vi "Process serial data.vi"(5 "Data in":string="SRNO=23234\nSOFT=40316\nXRT1=109\nSTAT=1089\nFREQ=170000\nSYNC=12345678\nEPOS=0\nDPOS=0\nINFO=2\nTIME=8427") -> (0 "Stage types":string[][](array[string]), 1 "Values":i32[](array[numeric]), 2 "Parameters":T1[](array[typedef]), 3 "Drive letters":string[](array[string]))   [LabVIEW 2019]
uses:
  Class/Controller/Serial parameters.ctl
  Class/Controller/Controller.lvclass
panel:
  out "array":string[](array[string])
  # "Example data single axis"
  # "Example data multi axis"
  # "SRNO=23234\nSOFT=40316\nXRT1=109\nSTAT=1089\nFREQ=170000\nSYNC=12345678\nEPOS=0\nDPOS=0\nINFO=2\nTIME=8427"
  # "A:SRNO=0\nA:SOFT=40305\nA:XLS1=313\nA:STAT=17\nA:FREQ=170000\nA:SYNC=12345678\nA:EPOS=2\nA:DPOS=0\nA:PHAC=0\nA:TIME=55599\nB:SRNO=0\nB:SOFT=40305\nB:XLA1=312\nB:STAT=17\nB:FREQ=173000\nB:SYNC=12345678\nB:EPOS=1\nB:DPOS=0\nB:PROP=120\nB:TIME=29533\nC:SRNO=0\nC:SOFT=40305\nC:XRT1=109\nC:STAT=1\nC:FREQ=173000\nC:SYNC=12345678\nC:EPOS=0\nC:DPOS=0\nC:PROP=120\nC:TIME=30364\nD:SRNO=0\nD:SOFT=40305\nD:XLS3=1251\nD:STAT=401\nD:FREQ=87000\nD:SYNC=12345678\nD:EPOS=0\nD:DPOS=0\nD:PROP=120\nD:TIME=30387\nE:SRNO=0\nE:SOFT=40305\nE:XLA3=1250\nE:STAT=17\nE:FREQ=87000\nE:SYNC=12345678\nE:EPOS=0\nE:DPOS=0\nE:PROP=120\nE:TIME=30355"
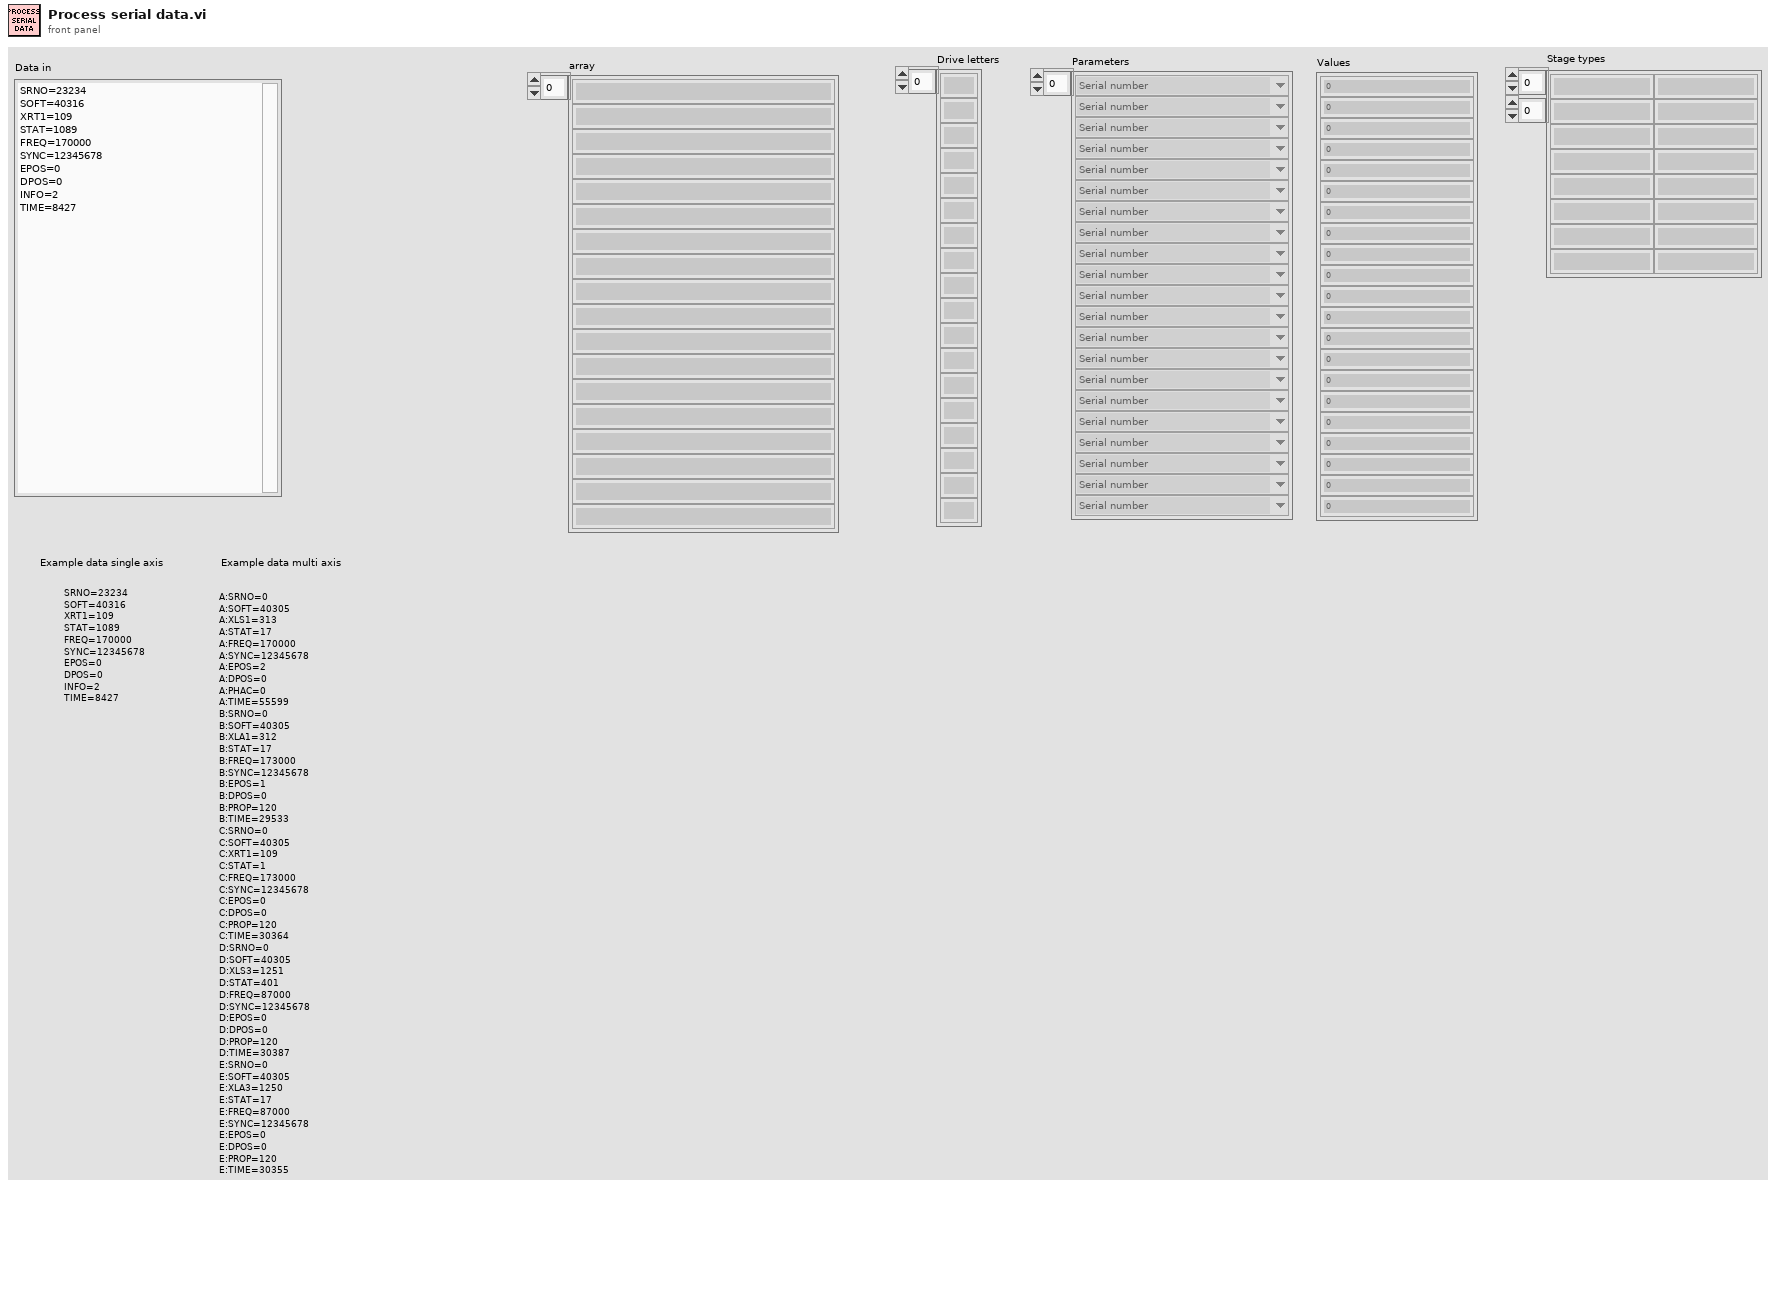
[diagram p1: front panel]
types:
  T1 = typedef "Controller.lvclass/Serial parameters.ctl" = enum16{"Serial number", "Software number", "Type of stage", "Status", "Frequency", "Encoder position", "Desired position", "Info", "Phase correction", "Timestamp", "Proportional control factor", "Sync", "XRT1", "XRT3", "XRTA", "XLS1", "XLS3", "XLA1", "XLA3"}
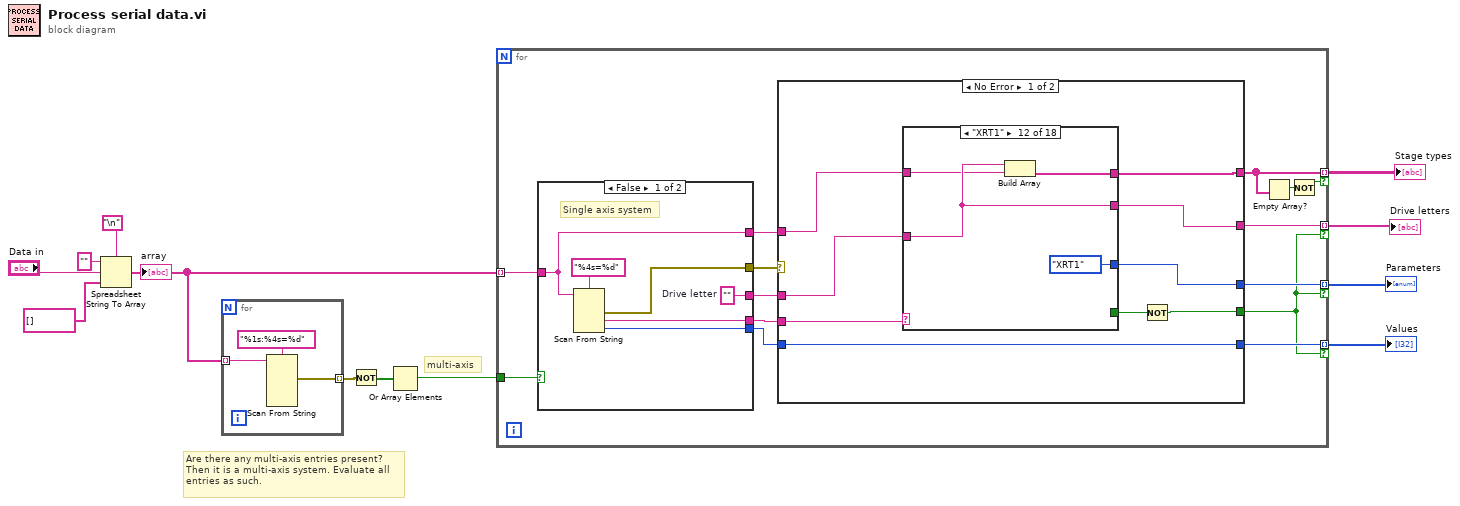
[diagram p0: block diagram]
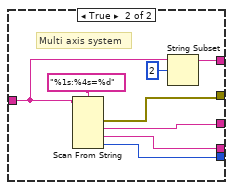
[diagram p2: hidden frame]
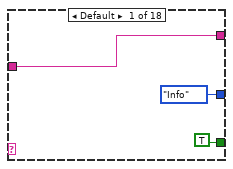
[diagram p3: hidden frame]
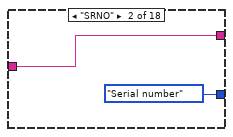
[diagram p4: hidden frame]
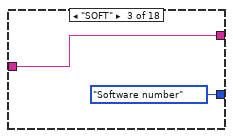
[diagram p5: hidden frame]
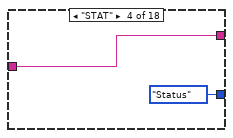
[diagram p6: hidden frame]
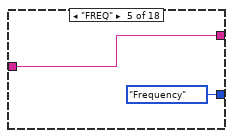
[diagram p7: hidden frame]
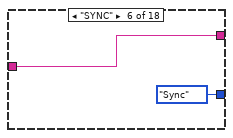
[diagram p8: hidden frame]
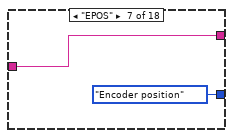
[diagram p9: hidden frame]
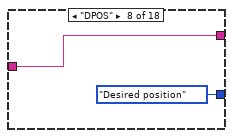
[diagram p10: hidden frame]
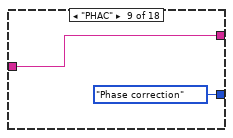
[diagram p11: hidden frame]
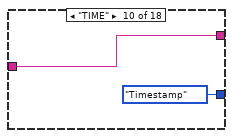
[diagram p12: hidden frame]
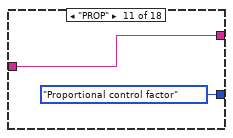
[diagram p13: hidden frame]
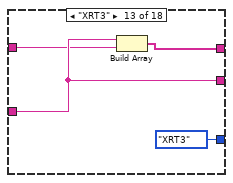
[diagram p14: hidden frame]
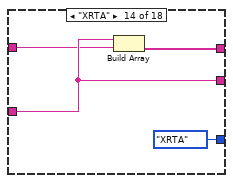
[diagram p15: hidden frame]
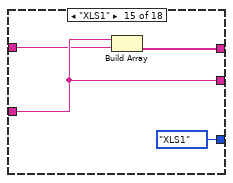
[diagram p16: hidden frame]
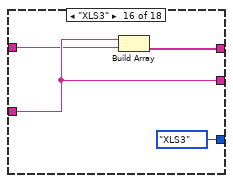
[diagram p17: hidden frame]
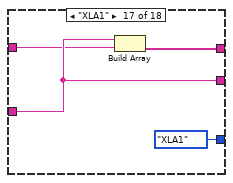
[diagram p18: hidden frame]
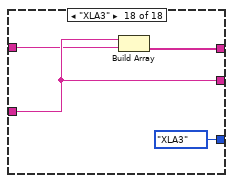
[diagram p19: hidden frame]
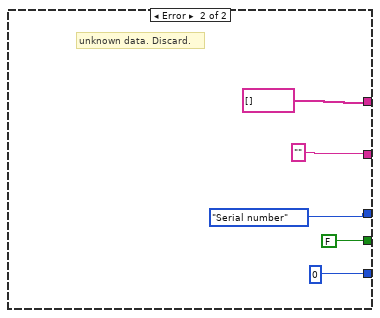
[diagram p20: hidden frame]
diagram:
  # "multi-axis"
  # "Are there any multi-axis entries present?\nThen it is a multi-axis system. Evaluate all\nentries as such."
  n1 = Spreadsheet String To Array(delimiter (Tab)="\n", format string="", spreadsheet string="Data in", array type (2D Dbl)=string[] []) -> (array=w4:string[])
  "array" <- w4
  n2 = for {
    tunnel: w4 -> [w14] mode=indexing
    tunnel: [w13] -> w3 mode=indexing
    n3 = Scan From String(format string="%1s:%4s=%d", input string=w14) -> (error out=w13:errorcluster)  [unwired: 8 in, 2 out]
  }
  n4 = Not(x=w3) -> (.not. x?=w2:bool[])
  n5 = Or Array Elements(Boolean array=w2) -> (logical OR=w1:bool)
  n6 = for {
    tunnel: w4 -> [w27] mode=indexing
    tunnel: [w29] -> w8 mode=indexing if=w22
    tunnel: [w28] -> w7 mode=indexing if=w22
    tunnel: [w23] -> w6 mode=indexing if=w22
    tunnel: [w21] -> w5 mode=indexing if=w19
    tunnel: w1 -> [w18]
    n7 = case shown="False" w18 {
      tunnel: w27 -> [w30 w38]
      tunnel: [w34 w40] -> w26
      tunnel: [w33 w39] -> w25
      tunnel: [w32 w42] -> w24
      tunnel: [w31 w41] -> w17
      tunnel: [w30 w36] -> w16
      frame False {
        w31 = ""  # Drive letter
        # "Single axis system"
        n8 = Scan From String(format string="%4s=%d", input string=w30) -> (error out=w32:errorcluster, output 1=w34:string, output 2=w33:i32)  [unwired: 4 in, 2 out]
      }
      frame True {
        # "Multi axis system"
        n9 = Scan From String(format string="%1s:%4s=%d", input string=w38) -> (error out=w42:errorcluster, output 1=w41:string, output 2=w40:string, output 3=w39:i32)  [unwired: 5 in, 2 out]
        n10 = String Subset(string=w38, offset (0)=2) -> (substring=w36:string)  [unwired: 1 in]
      }
    }
    n11 = case shown="No Error" w24 {
      tunnel: [w45 Serial_parameters."Serial number" ("Enum")] -> w29
      tunnel: [w52 0] -> w28
      tunnel: [w44 FALSE] -> w22
      tunnel: [w47 string[] [] ("Stage types")] -> w21
      tunnel: w16 -> [w49 _]
      tunnel: w26 -> [w48 _]
      tunnel: w25 -> [w52 _]
      tunnel: [w46 ""] -> w23
      tunnel: w17 -> [w50 _]
      frame No Error {
        n12 = case shown="\"XRT1\"" w48 {
          tunnel: [Serial_parameters."Info" ("Enum") Serial_parameters."Serial number" ("Enum") Serial_parameters."Software number" ("Enum") Serial_parameters."Status" ("Enum") Serial_parameters."Frequency" ("Enum") Serial_parameters."Sync" ("Enum") Serial_parameters."Encoder position" ("Enum") Serial_parameters."Desired position" ("Enum") Serial_parameters."Phase correction" ("Enum") Serial_parameters."Timestamp" ("Enum") Serial_parameters."Proportional control factor" ("Enum") Serial_parameters."XRT1" ("Enum") Serial_parameters."XRT3" ("Enum") Serial_parameters."XRTA" ("Enum") Serial_parameters."XLS1" ("Enum") Serial_parameters."XLS3" ("Enum") Serial_parameters."XLA1" ("Enum") Serial_parameters."XLA3" ("Enum")] -> w45
          tunnel: [TRUE _ _ _ _ _ _ _ _ _ _ _ _ _ _ _ _ _] -> w51
          tunnel: w49 -> [_ _ _ _ _ _ _ _ _ _ _ w77 w81 w85 w89 w93 w97 w101]
          tunnel: [w53 w56 w58 w60 w62 w64 w66 w68 w70 w72 w74 w78 w82 w86 w90 w94 w98 w102] -> w46
          tunnel: w50 -> [w53 w56 w58 w60 w62 w64 w66 w68 w70 w72 w74 w78 w82 w86 w90 w94 w98 w102]
          tunnel: [_ _ _ _ _ _ _ _ _ _ _ w76 w80 w84 w88 w92 w96 w100] -> w47
          frame Default {
          }
          frame "SRNO" {
          }
          frame "SOFT" {
          }
          frame "STAT" {
          }
          frame "FREQ" {
          }
          frame "SYNC" {
          }
          frame "EPOS" {
          }
          frame "DPOS" {
          }
          frame "PHAC" {
          }
          frame "TIME" {
          }
          frame "PROP" {
          }
          frame "XRT1" {
            n13 = Build Array(w78, w77) -> (w76:string[])
          }
          frame "XRT3" {
            n14 = Build Array(w82, w81) -> (w80:string[])
          }
          frame "XRTA" {
            n15 = Build Array(w86, w85) -> (w84:string[])
          }
          frame "XLS1" {
            n16 = Build Array(w90, w89) -> (w88:string[])
          }
          frame "XLS3" {
            n17 = Build Array(w94, w93) -> (w92:string[])
          }
          frame "XLA1" {
            n18 = Build Array(w98, w97) -> (w96:string[])
          }
          frame "XLA3" {
            n19 = Build Array(w102, w101) -> (w100:string[])
          }
        }
        n20 = Not(x=w51) -> (.not. x?=w44:bool)
      }
      frame Error {
        # "unknown data. Discard."
      }
    }
    n21 = Empty Array?(array=w21) -> (empty?=w20:bool)
    n22 = Not(x=w20) -> (.not. x?=w19:bool)
  }
  "Parameters" <- w8
  "Values" <- w7
  "Drive letters" <- w6
  "Stage types" <- w5
